vi "Calc X from V_out.vi"(0 "Ta (°C)":dbl=25.0, 1 "Overheat ratio (Rw / R0)":dbl=1.7, 2 "Gain":dbl=17.466666666666665, 3 "Offset (V)":dbl=0.512, 4 "alpha0 (/°C)":dbl=0.0036, 5 "Bridge ratio":dbl=1.0, 6 "V_out (V)":dbl=3.85584, 7 "R0 (ohm)":dbl=3.5, 9 "RL (ohm)":dbl=0.5, 11 "Wire length (m)":dbl=0.00125, 13 "T0 (°C)":dbl=20.0) -> (14 "X":dbl=1.0000020231248197)   [LabVIEW 2022 SP3]
doc: "Calculate X from V_out (taking into account Ta).\nPN 05-NOV-23."
panel:
  # "V_out = G * (V_bridge - V_offset)"
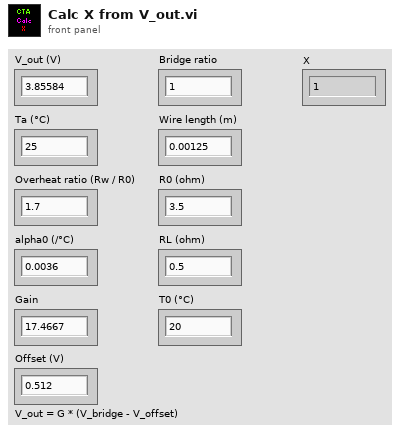
[diagram p1: front panel]
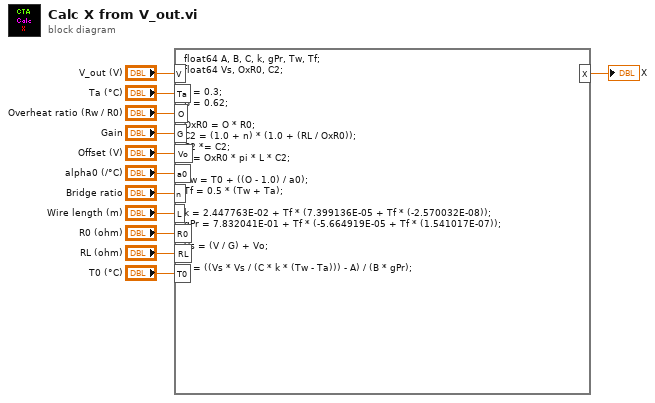
[diagram p0: block diagram]
diagram:
  n1 = formula code="float64 A, B, C, k, gPr, Tw, Tf;\nfloat64 Vs, OxR0, C2;\n\nA = 0.3;\nB = 0.62;\n\nOxR0 = O * R0;\nC2 = (1.0 + n) * (1.0 + (RL / OxR0));\nC2 *= C2;\nC = OxR0 * pi * L * C2;\n\nTw = T0 + ((O - 1.0) / a0);\nTf = 0.5 * (Tw + Ta);\n\nk = 2.447763E-02 + Tf * (7.399136E-05 + Tf * (-2.570032E-08));\ngPr = 7.832041E-01 + Tf * (-5.664919E-05 + Tf * (1.541017E-07));\n\nVs = (V / G) + Vo;\n\nX = ((Vs * Vs / (C * k * (Tw - Ta))) - A) / (B * gPr);"("V"="V_out (V)", "Ta"="Ta (°C)", "O"="Overheat ratio (Rw / R0)", "a0"="alpha0 (/°C)", "n"="Bridge ratio", "L"="Wire length (m)", "R0"="R0 (ohm)", "RL"="RL (ohm)", "T0"="T0 (°C)", "G"="Gain", "Vo"="Offset (V)") -> ("X"=→"X":dbl)
